vi "SampleMaster.vi"() -> ()   [LabVIEW 2016]
doc: "A sample master that can be run on the computer or RIO"
panel:
  out "ms/it":u32(graph)
  out "iteration":i32
  in  "Service call":bool
  in  "Show Web":bool
  in  "Show Node":bool
  out "Answer":string
  in  "LED":bool
  out "LED reply":string
  out "time":string
  out "Status":string
  in  "stop":bool
  # "Instructions:\n1. Run the VI\n2. Verify that you see the correct time.\n3. Press the LED button. You should see the LED reply change.\nIf you are targetting a myRIO, the LED should change as well.\n4. Debug by clicking Show Node and Show Webpage.\n5. See what is being sent back and forth by clicking Show Node and Show Webpage."
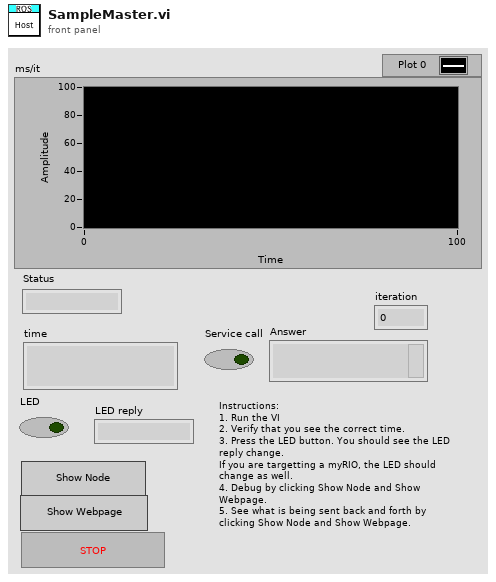
[diagram p1: front panel]
types:
  T1 = typedef "_ROSControl.ctl" = cluster{"topic port":u16, "Node":string, "topic":string, "type":string, "node port":u16, "error ":errorcluster, "Direction":T2, "Update (ms)":u16, "FIFO size":u16}
  T2 = typedef "_ROSDirection.ctl" = enum16{"Node", "Publisher", "Subscriber", "ServiceClient", "ServiceProvider"}
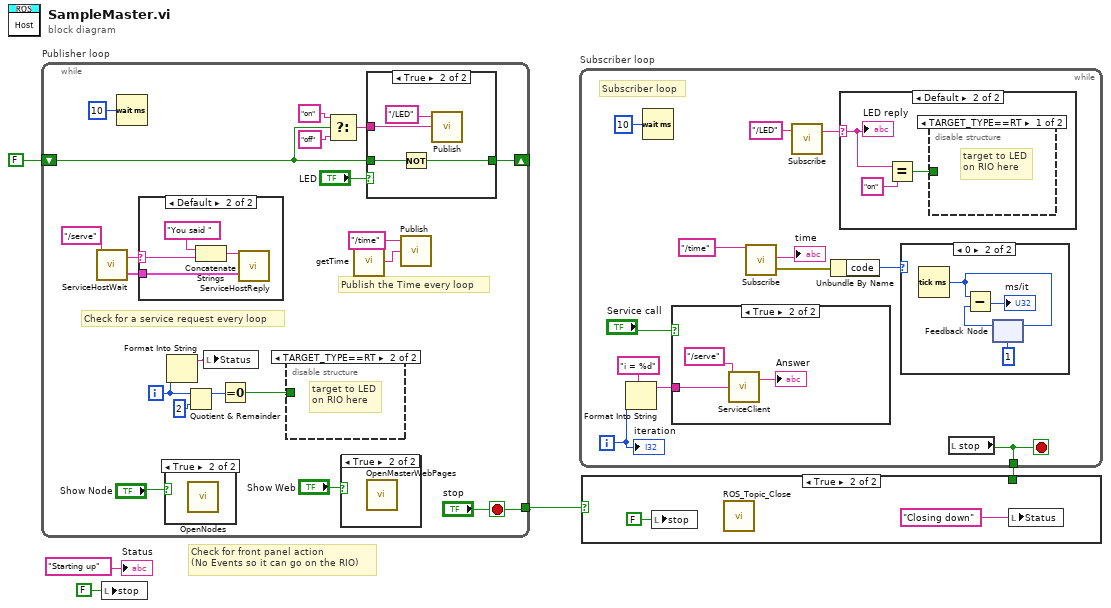
[diagram p0: block diagram]
diagram:
  # "Check for front panel action\n(No Events so it can go on the RIO)"
  n1 = while "Publisher loop" {
    tunnel: ["stop"] -> w3
    shift-right: [w21] -> _
    shift-left: FALSE -> [w20]
    i -> [w12]
    stop <- "stop" stop-if-true
    # "Check for a service request every loop"
    # "Publish the Time every loop"
    n2 = call "ServiceHostWait.vi"("Topic"="/serve") -> ("Request"=w6:string, "Service ROS info out"=w8:T1)  [unwired: 4 in]
    n3 = Wait (ms)(milliseconds to wait=u32 10) -> ()  [unwired: 1 out]
    n4 = case shown="Default" w6 {
      selector: w6 -> [_ w26]
      tunnel: w8 -> [_ w28]
      frame "" {
      }
      frame Default {
        n5 = Concatenate Strings("You said " ("string"), w26) -> (w27:string)
        n6 = call "ServiceHostReply.vi"("Service ROS info in"=w28, "Reply"=w27) -> ()  [unwired: 2 in, 1 out]
      }
    }
    n7 = case shown="True" "Show Node" {
      frame False {
      }
      frame True {
        n8 = call "OpenNodes.vi"() -> ()  [unwired: 2 in]
      }
    }
    n9 = Format Into String(w12) -> (resulting string=w25:string)  [unwired: 3 in, 1 out]
    n10 = Quotient & Remainder(x=w12, y=2) -> (x-y*floor(x/y)=w14:i32)  [unwired: 1 out]
    n11 = local write "Status"(w25) -> ()
    n12 = Equal To 0?(x=w14) -> (x = 0?=w13:bool)
    n13 = disable-structure shown="TARGET_TYPE==RT" {
      disable-tunnel: w13 -> [_ _]
      frame condition #0 {
      }
      frame condition #1 (active) {
        # "target to LED\non RIO here"
      }
    }
    n14 = Select(t="on" ("Status"), s=w20, f="off" ("Status")) -> (s? t:f=w22:string)
    n15 = case shown="True" "Show Web" {
      frame False {
      }
      frame True {
        n16 = call "OpenMasterWebPages.vi"() -> ()  [unwired: 4 in]
      }
    }
    n17 = call "getTime.vi"() -> ("Current Time"=w10:string)  [unwired: 1 in]
    n18 = case shown="True" "LED" {
      tunnel: w22 -> [_ w32]
      tunnel: [w30 w33] -> w21
      tunnel: w20 -> [w30 w34]
      frame False {
      }
      frame True {
        n19 = Not(x=w34) -> (.not. x?=w33:bool)
        n20 = call "Publish.vi"("Topic"="/LED", "String"=w32) -> ()  [unwired: 5 in, 1 out]
      }
    }
    n21 = call "Publish.vi"("Topic"="/time", "String"=w10) -> ()  [unwired: 5 in, 1 out]
  }
  n22 = local write "stop"(FALSE ("stop")) -> ()
  n23 = while "Subscriber loop" {
    tunnel: [w40] -> w2
    i -> [w44]
    stop <- w40 stop-if-true
    # "Subscriber loop"
    n24 = Format Into String(format string="i = %d" ("Msg in"), w44) -> (resulting string=w43:string)  [unwired: 2 in, 1 out]
    n25 = Wait (ms)(milliseconds to wait=u32 10) -> ()  [unwired: 1 out]
    n26 = case shown="True" "Service call" {
      tunnel: w43 -> [_ w55]
      frame False {
      }
      frame True {
        n27 = call "ServiceClient.vi"("Topic"="/serve", "Msg in"=w55) -> ("Reply"=→"Answer":string)  [unwired: 3 in, 1 out]
      }
    }
    n28 = call "Subscribe.vi"("Topic"="/time") -> ("error out"=w38:errorcluster, "Reply"=→"time":string)  [unwired: 2 in]
    n29 = call "Subscribe.vi"("Topic"="/LED") -> ("Reply"=w42:string)  [unwired: 2 in, 1 out]
    n30 = Unbundle By Name(w38) -> ("code"=w39:i32)
    n31 = case shown="Default" w42 {
      selector: w42 -> [_ w53]
      frame "" {
      }
      frame Default {
        n32 = Equal?(x=w53, y="on" ("Status")) -> (x = y?=w51:bool)
        n33 = disable-structure shown="TARGET_TYPE==RT" {
          disable-tunnel: w51 -> [_ _]
          frame condition #0 (active) {
            # "target to LED\non RIO here"
          }
          frame condition #1 {
          }
        }
        "LED reply" <- w53
      }
    }
    n34 = case shown="0" w39 {
      frame Default {
      }
      frame 0 {
        n35 = Tick Count (ms)() -> (millisecond timer value=w49:u32)
        n36 = feedback-in #1(w49) -> ()
        n37 = feedback #1(u32 1 ("milliseconds to wait")) -> (w48:u32)
        n38 = Subtract(x=w49, y=w48) -> (x-y=→"ms/it":u32)
      }
    }
    n39 = local read "stop"() -> (w40:bool)
    "iteration" <- w44
  }
  n40 = case shown="True" w3 {
    tunnel: w2 -> [_ _]
    frame False {
    }
    frame True {
      n41 = local write "stop"(FALSE ("stop")) -> ()
      n42 = call "ROS_Topic_Close.vi"() -> ()  [unwired: 4 in, 1 out]
      n43 = local write "Status"("Closing down" ("Status")) -> ()
    }
  }
  "Status" <- "Starting up" ("Status")
